vi "Read Section Temp.vi"(0 "section":string="S1") -> (4 "Data Cluster":cluster{bool, "Tx":T1, "TxO":T2, "TxA":T3})   [LabVIEW 2017, in "Konfiguracja.lvlib"]
uses:
  Konfiguracja/Konfiguracja.lvlib
  SupportVIs/Konfiguracja/Controls/TxA.ctl
  SupportVIs/Konfiguracja/Controls/TxO.ctl
  SupportVIs/Konfiguracja/Controls/Tx.ctl
  <vilib>/Utility/config.llb/NI_LVConfig.lvlib
panel:
  in  "Tx":T1
  in  "TxO":T2
  in  "TxA":T3
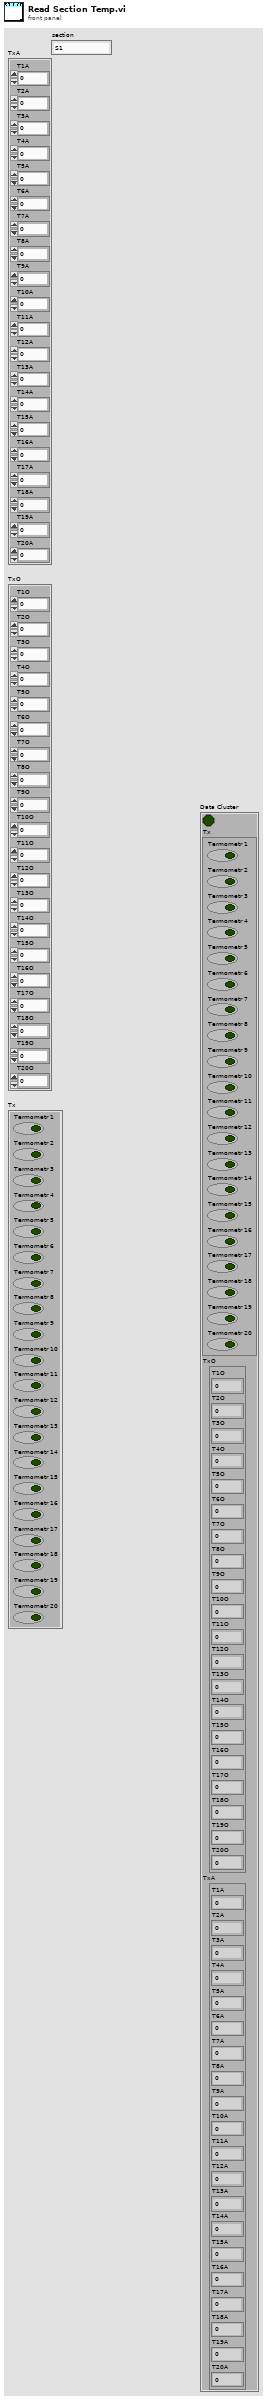
[diagram p1: front panel]
types:
  T1 = typedef "Konfiguracja.lvlib/Tx.ctl" = cluster{"Termometr 1":bool, "Termometr 2":bool, "Termometr 3":bool, "Termometr 4":bool, "Termometr 5":bool, "Termometr 6":bool, "Termometr 7":bool, "Termometr 8":bool, "Termometr 9":bool, "Termometr 10":bool, "Termometr 11":bool, "Termometr 12":bool, "Termometr 13":bool, "Termometr 14":bool, "Termometr 15":bool, "Termometr 16":bool, "Termometr 17":bool, "Termometr 18":bool, "Termometr 19":bool, "Termometr 20":bool}
  T2 = typedef "Konfiguracja.lvlib/TxO.ctl" = cluster{"T1O":dbl, "T2O":dbl, "T3O":dbl, "T4O":dbl, "T5O":dbl, "T6O":dbl, "T7O":dbl, "T8O":dbl, "T9O":dbl, "T10O":dbl, "T11O":dbl, "T12O":dbl, "T13O":dbl, "T14O":dbl, "T15O":dbl, "T16O":dbl, "T17O":dbl, "T18O":dbl, "T19O":dbl, "T20O":dbl}
  T3 = typedef "Konfiguracja.lvlib/TxA.ctl" = cluster{"T1A":dbl, "T2A":dbl, "T3A":dbl, "T4A":dbl, "T5A":dbl, "T6A":dbl, "T7A":dbl, "T8A":dbl, "T9A":dbl, "T10A":dbl, "T11A":dbl, "T12A":dbl, "T13A":dbl, "T14A":dbl, "T15A":dbl, "T16A":dbl, "T17A":dbl, "T18A":dbl, "T19A":dbl, "T20A":dbl}
  T4 = typedef "NI_LVConfig.lvlib/Config Data RefNum.ctl" = refnum<k1>
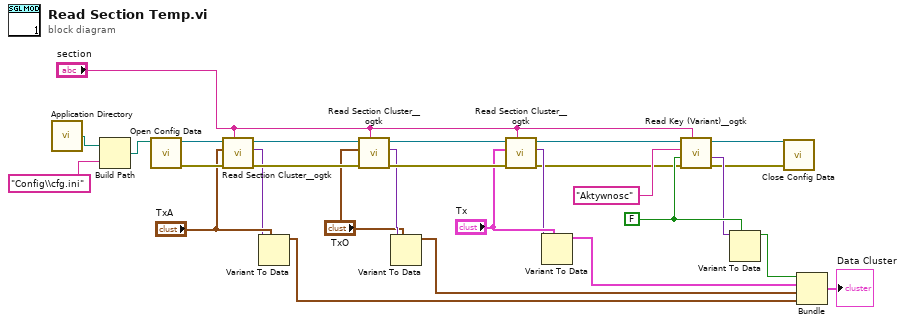
[diagram p0: block diagram]
diagram:
  w9 = FALSE
  n1 = call <vilib>:"Application Directory.vi"() -> ("Application Directory"=w15:path)
  n2 = Build Path(base path=w15, name or relative path="Config\\cfg.ini") -> (appended path=w17:path)
  n3 = call <vilib>:"Open Config Data.vi"("configuration file path"=w17) -> ("error out"=w26:errorcluster, "refnum"=w11:T4)  [unwired: 8 in, 1 out]
  n4 = call <userlib>:"Read Section Cluster__ogtk.vi"("section (optional)"="section", "error in (no error)"=w26, "Section Formatted Cluster Type"="TxA", "refnum"=w11) -> ("error out"=w27:errorcluster, "Section Formatted Cluster"=w20:variant, "dup refnum"=w18:T4)  [unwired: 3 in, 2 out]
  n5 = Variant To Data(type="TxA", Variant=w20) -> (data=w14:T3)  [unwired: 1 in, 1 out]
  n6 = call <userlib>:"Read Section Cluster__ogtk.vi"("section (optional)"="section", "error in (no error)"=w27, "Section Formatted Cluster Type"="TxO", "refnum"=w18) -> ("error out"=w28:errorcluster, "Section Formatted Cluster"=w23:variant, "dup refnum"=w19:T4)  [unwired: 3 in, 2 out]
  n7 = Variant To Data(type="TxO", Variant=w23) -> (data=w13:T2)  [unwired: 1 in, 1 out]
  n8 = call <userlib>:"Read Section Cluster__ogtk.vi"("section (optional)"="section", "error in (no error)"=w28, "Section Formatted Cluster Type"="Tx", "refnum"=w19) -> ("error out"=w5:errorcluster, "Section Formatted Cluster"=w24:variant, "dup refnum"=w6:T4)  [unwired: 3 in, 2 out]
  n9 = Variant To Data(type="Tx", Variant=w24) -> (data=w12:T1)  [unwired: 1 in, 1 out]
  n10 = call <userlib>:"Read Key (Variant)__ogtk.vi"("section"="section", "error in (no error)"=w5, "type"=w9, "key (optional)"="Aktywnosc", "refnum"=w6) -> ("error out"=w2:errorcluster, "key-value"=w8:variant, "refnum out"=w3:T4)  [unwired: 3 in, 1 out]
  n11 = Variant To Data(type=w9, Variant=w8) -> (data=w4:bool)  [unwired: 1 in, 1 out]
  n12 = call <vilib>:"Close Config Data.vi"("error in (no error)"=w2, "refnum"=w3) -> ()  [unwired: 8 in, 2 out]
  n13 = Bundle(w4, "Tx"=w12, "TxO"=w13, "TxA"=w14) -> (→"Data Cluster":cluster{bool, "Tx":T1, "TxO":T2, "TxA":T3})  [unwired: 1 in]
